vi "Scan_SetGraphScales.vi"(8 "error in (no error)":errorcluster, 10 "Image Measurent Parameters":T1, 11 "Image":refnum<vi>) -> (0 "error out":errorcluster)   [LabVIEW 2009]
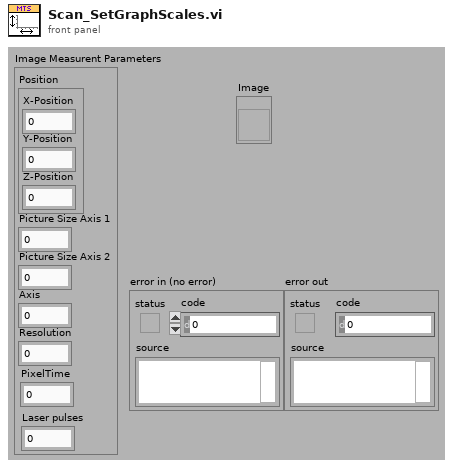
[diagram p1: front panel]
types:
  T1 = cluster{"Position":cluster{"X-Position":dbl, "Y-Position":dbl, "Z-Position":dbl}, "Picture Size Axis 1":dbl, "Picture Size Axis 2":dbl, "Axis":i32, "Resolution":dbl, "PixelTime":dbl, "Laser pulses":i32}
  T2 = cluster{"X-Position":dbl, "Y-Position":dbl, "Z-Position":dbl}
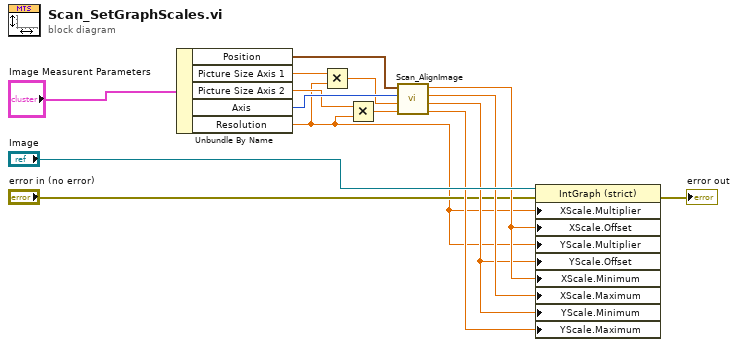
[diagram p0: block diagram]
diagram:
  n1 = Unbundle By Name("Image Measurent Parameters") -> ("Position"=w12:T2, "Picture Size Axis 1"=w11:dbl, "Picture Size Axis 2"=w2:dbl, "Axis"=w10:i32, "Resolution"=w1:dbl)
  n2 = Multiply(x=w11, y=w1) -> (x*y=w3:dbl)
  n3 = Multiply(x=w2, y=w1) -> (x*y=w4:dbl)
  n4 = call "Scan_AlignImage.vi"("slow axis"=w4, "fast axis"=w3, "Axis"=w10, "Scanner XYZ"=w12) -> ("Image Y end"=w8:dbl, "Image Y start"=w6:dbl, "Image X end"=w9:dbl, "Image X start"=w7:dbl)  [unwired: 1 in]
  n5 = property on="Property Node" class="IntGraph (strict)"(reference="Image", error in="error in (no error)", "XScale.Multiplier"=w1, "XScale.Offset"=w7, "YScale.Multiplier"=w1, "YScale.Offset"=w6, "XScale.Minimum"=w7, "XScale.Maximum"=w9, "YScale.Minimum"=w6, "YScale.Maximum"=w8) -> (error out=→"error out":errorcluster)  [unwired: 1 out]
